vi "RP EEPROM to Scale.vi"(6 "Signal bits":i32=14, 9 "Ranges":dbl[](array[numeric]), 11 "EEPROM calibration":T1 {"magic" format="%x"}) -> (1 "Magic?":bool, 2 "Scaling coefficients":dbl[][](array[numeric]))   [LabVIEW 2018]
uses:
  RP EEPROM Calibration.ctl
panel:
  in  "Channel":i32
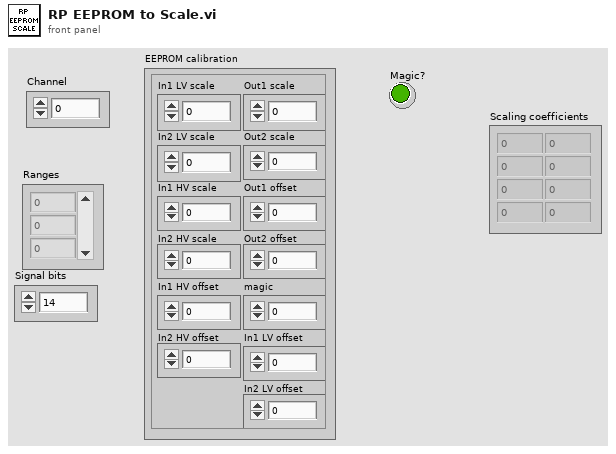
[diagram p1: front panel]
types:
  T1 = typedef "RP EEPROM Calibration.ctl" = cluster{"In1 LV scale":u32, "In2 LV scale":u32, "In1 HV scale":u32, "In2 HV scale":u32, "In1 HV offset":i32, "In2 HV offset":i32, "Out1 scale":u32, "Out2 scale":u32, "Out1 offset":i32, "Out2 offset":i32, "magic":u32, "In1 LV offset":i32, "In2 LV offset":i32}
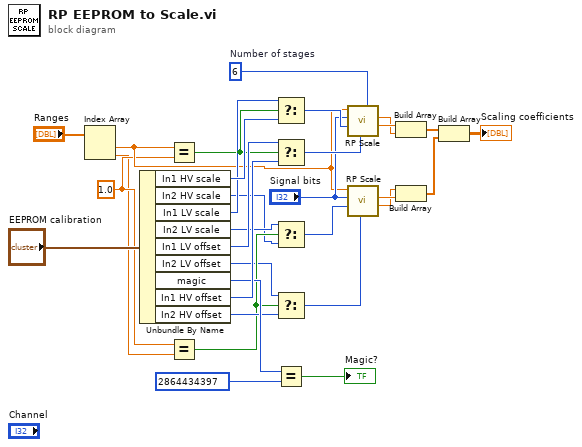
[diagram p0: block diagram]
diagram:
  w23 = 6  # Number of stages
  w6 = 1.0 ("y")
  n1 = Index Array(array="Ranges") -> (element #1=w7:dbl, element #2=w5:dbl)  [unwired: 2 in]
  n2 = Unbundle By Name("EEPROM calibration") -> ("In1 HV scale"=w31:u32, "In2 HV scale"=w2:u32, "In1 LV scale"=w30:u32, "In2 LV scale"=w3:u32, "In1 LV offset"=w29:i32, "In2 LV offset"=w1:i32, "magic"=w27:u32, "In1 HV offset"=w28:i32, "In2 HV offset"=w18:i32)
  n3 = Equal?(x=w7, y=w6) -> (x = y?=w17:bool)
  n4 = Equal?(x=w6, y=w5) -> (x = y?=w4:bool)
  n5 = Select(t=w30, s=w17, f=w31) -> (s? t:f=w25:u32)
  n6 = Select(t=w29, s=w17, f=w28) -> (s? t:f=w24:i32)
  n7 = Select(t=w3, s=w4, f=w2) -> (s? t:f=w21:u32)
  n8 = Select(t=w1, s=w4, f=w18) -> (s? t:f=w16:i32)
  n9 = Equal?(x=w27, y=u32 2864434397) -> (x = y?=→"Magic?":bool)
  n10 = call "RP Scale.vi"("Number of stages"=w23, "EEPROM offset"=w24, "EEPROM range"=w25, "Signal bits"="Signal bits", "Range"=w7) -> ("y intersept"=w11:dbl, "Calibrated slope"=w10:dbl)  [unwired: 4 in, 1 out]
  n11 = call "RP Scale.vi"("EEPROM offset"=w16, "EEPROM range"=w21, "Signal bits"="Signal bits", "Range"=w7) -> ("y intersept"=w8:dbl, "Calibrated slope"=w9:dbl)  [unwired: 5 in, 1 out]
  n12 = Build Array(w11, w10) -> (w14:dbl[])
  n13 = Build Array(w8, w9) -> (w13:dbl[])
  n14 = Build Array(w14, w13) -> (→"Scaling coefficients":dbl[][])
